vi "Write CCD Config to Header.vi"(8 "error in (no error)":errorcluster, 10 "CCD Config":T1, 11 "Header in":refnum<class "Simulated_Header.lvclass">) -> (0 "error out":errorcluster, 3 "Header out":refnum<class "Simulated_Header.lvclass">)   [LabVIEW 2018, in "Simulated_Header.lvclass"]
uses:
  Simulated_Header.lvclass
  Simulated_Header.lvclass/Simulated_Header.ctl
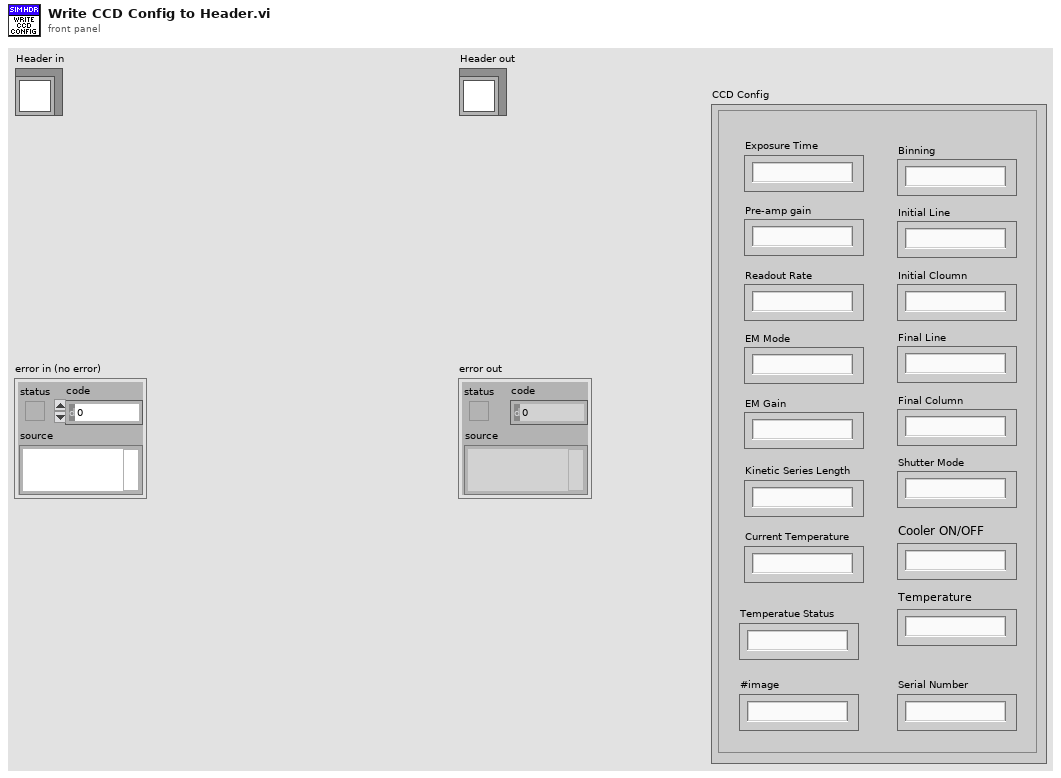
[diagram p1: front panel]
types:
  T1 = cluster{"Exposure Time":string, "Pre-amp gain":string, "Readout Rate":string, "EM Mode":string, "EM Gain":string, "Binning":string, "Initial Line":string, "Initial Cloumn":string, "Final Line":string, "Final Column":string, "Kinetic Series Length":string, "Shutter Mode":string, "Cooler ON/OFF":string, "Temperature":string, "Current Temperature":string, "Temperatue Status":string, "Serial Number":string, "#image":string}
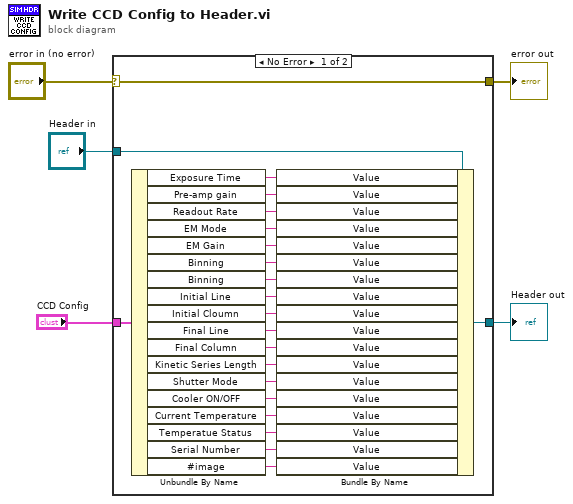
[diagram p0: block diagram]
diagram:
  n1 = case shown="No Error" "error in (no error)" {
    selector: "error in (no error)" -> [w27 w29]
    tunnel: [w27 w29] -> w4
    tunnel: [w7 w28] -> w2
    tunnel: "Header in" -> [w26 w28]
    tunnel: "CCD Config" -> [w25 _]
    frame No Error {
      n2 = Unbundle By Name(w25) -> ("Exposure Time"=w24:string, "Pre-amp gain"=w23:string, "Readout Rate"=w22:string, "EM Mode"=w8:string, "EM Gain"=w9:string, "Binning"=w21:string, "Binning"=w10:string, "Initial Line"=w11:string, "Initial Cloumn"=w12:string, "Final Line"=w13:string, "Final Column"=w14:string, "Kinetic Series Length"=w15:string, "Shutter Mode"=w20:string, "Cooler ON/OFF"=w16:string, "Current Temperature"=w17:string, "Temperatue Status"=w18:string, "Serial Number"=w19:string, "#image"=w6:string)
      n3 = Bundle By Name(cluster=w26, "Value"=w24, "Value"=w23, "Value"=w22, "Value"=w8, "Value"=w9, "Value"=w21, "Value"=w10, "Value"=w11, "Value"=w12, "Value"=w13, "Value"=w14, "Value"=w15, "Value"=w20, "Value"=w16, "Value"=w17, "Value"=w18, "Value"=w19, "Value"=w6) -> (w7:refnum<class "Simulated_Header.lvclass">)
    }
    frame Error {
    }
  }
  "error out" <- w4
  "Header out" <- w2
